vi "Terminate Test.vi"(8 "error in (no error)":errorcluster, 11 "PLC_Module in":refnum<class "PLC_Module.lvclass">) -> (0 "error out":errorcluster, 3 "PLC_Module out":refnum<class "PLC_Module.lvclass">)   [LabVIEW 2025, in "PLC_Module.lvlib" / "PLC_Module.lvclass"]
uses:
  PLC_Module.lvclass
  PLC_Module.lvclass/PLC_Module.ctl
  4bd37e12-4a36-4441-ae7d-393c99274c78.vi
  Read Configuration.vi
  <vilib>/JDP Science/JSONtext/JSON text to Variant.vi
  <vilib>/Test Bench Framework/Terminate(Context).vi
  <vilib>/JDP Science/JSONtext/LVClass Serializer/JSONtext LVClass Serializer.lvclass
  <userlib>/_OpenG.lib/boolean/boolean.llb/openg_boolean__ogtk.lvlib
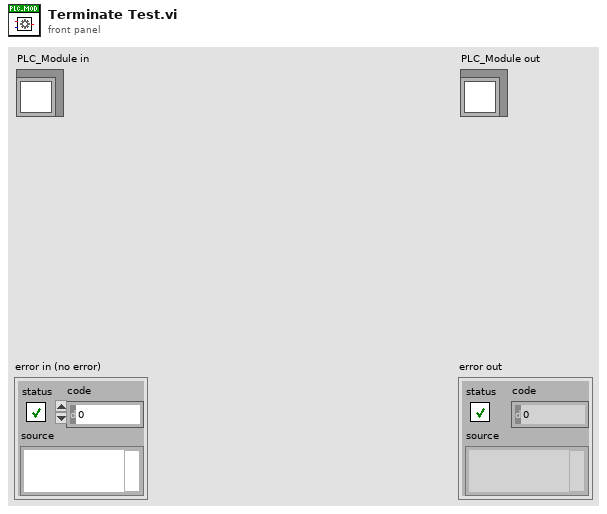
[diagram p1: front panel]
types:
  T1 = typedef "PLC_Module.lvlib/PLC_Module.lvclass/PLC_Data_Config.ctl" = map{string, cluster{"Config":T2, "Get Value":string, "Set Value":string}}
  T2 = typedef "PLC_Module.lvlib/PLC_Module.lvclass/PLC_Data.ctl" = cluster{"Address":string, "Direction":enum16{"PC->PLC", "PLC->PC"}, "DataType":T3, "Description":string}
  T3 = typedef "PLC_Module.lvlib/PLC_Module.lvclass/PLC_Data_Type.ctl" = enum16{"Boolean", "Single Float", "U8", "U32", "U32_Array", "String"}
  T4 = cluster{"Config":T2, "Get Value":string, "Set Value":string}
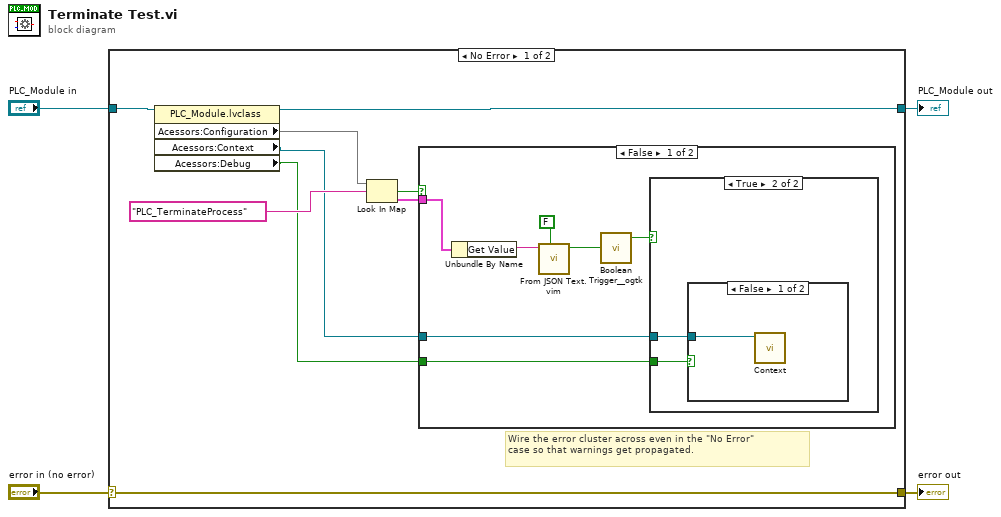
[diagram p0: block diagram]
diagram:
  n1 = case shown="No Error" "error in (no error)" {
    selector: "error in (no error)" -> [w13 w25]
    tunnel: [w13 w25] -> w3
    tunnel: [w7 w24] -> w1
    tunnel: "PLC_Module in" -> [w12 w24]
    frame No Error {
      # "Wire the error cluster across even in the \"No Error\"\ncase so that warnings get propagated."
      n2 = property class="PLC_Module.lvclass"(reference=w12) -> (reference out=w7:refnum<class "PLC_Module.lvclass">, "Acessors:Configuration"=w8:T1, "Acessors:Context"=w6:refnum<vi>, "Acessors:Debug"=w5:bool)  [unwired: 1 in, 1 out]
      n3 = Look In Map(map=w8, key="PLC_TerminateProcess") -> (key not found?=w9:bool, value=w10:T4)  [unwired: 1 in]
      n4 = case shown="False" w9 {
        tunnel: w10 -> [w20 _]
        tunnel: w6 -> [w15 _]
        tunnel: w5 -> [w14 _]
        frame False {
          n5 = Unbundle By Name(w20) -> ("Get Value"=w19:string)
          n6 = call "From JSON Text.vim"("Data Type and Default Value"=FALSE, "JSON"=w19) -> ("Data out"=w17:bool)  [unwired: 8 in, 1 out]
          n7 = call <userlib>:"Boolean Trigger__ogtk.vi"("Boolean Input"=w17) -> ("Rising Edge"=w16:bool)  [unwired: 1 in, 1 out]
          n8 = case shown="True" w16 {
            tunnel: w15 -> [_ w22]
            tunnel: w14 -> [_ w21]
            frame False {
            }
            frame True {
              n9 = case shown="False" w21 {
                tunnel: w22 -> [w23 _]
                frame False {
                  n10 = call-poly <vilib>:"Context.vi"("Context"=w23) -> ()  [unwired: 10 in, 1 out]
                }
                frame True {
                }
              }
            }
          }
        }
        frame True {
        }
      }
    }
    frame Error {
    }
  }
  "error out" <- w3
  "PLC_Module out" <- w1
